vi "macro_NumCmd_Send_Array.vi"() -> ()   [LabVIEW 2019, in "Trajectory_Library.lvlib"]
uses:
  VI/numCmd_ObtainQueue_Array.vi
  Trajectory_Library.lvlib
panel:
  in  "Values":dbl[](array[numeric])
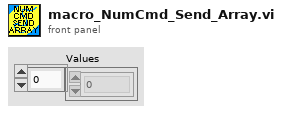
[diagram p1: front panel]
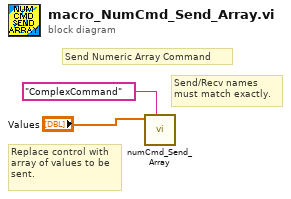
[diagram p0: block diagram]
diagram:
  # "Replace control with\narray of values to be \nsent."
  # "Send/Recv names\nmust match exactly."
  # "Send Numeric Array Command"
  n1 = call "numCmd_Send_Array.vi"("Command Name"="ComplexCommand", "Values"="Values") -> ()  [unwired: 9 in, 1 out]
